vi "Read Panel.vi"(8 "error in (no error)":errorcluster, 11 "Form Configuration in":refnum<class "Form Model Configuration.lvclass">) -> (0 "error out":errorcluster, 2 "Panel.lvlib:Panel.lvclass":refnum<class "Panel.lvclass">, 3 "Form Configuration out":refnum<class "Form Model Configuration.lvclass">)   [LabVIEW 2020]
uses:
  Form Model Configuration.lvclass
  <vilib>/MGI/Panel Manager/Panel/Panel/Panel.lvclass
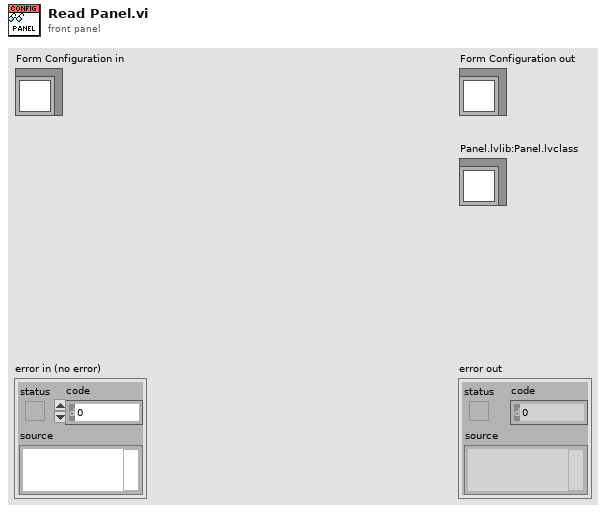
[diagram p1: front panel]
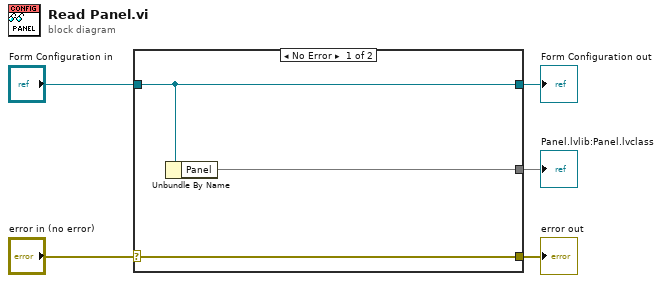
[diagram p0: block diagram]
diagram:
  n1 = case shown="No Error" "error in (no error)" {
    selector: "error in (no error)" -> [w8 w9]
    tunnel: [w8 w9] -> w4
    tunnel: [w7 w10] -> w2
    tunnel: "Form Configuration in" -> [w7 w10]
    tunnel: [w6 _] -> w1
    frame No Error {
      n2 = Unbundle By Name(w7) -> ("Panel"=w6)
    }
    frame Error {
    }
  }
  "error out" <- w4
  "Form Configuration out" <- w2
  "Panel.lvlib:Panel.lvclass" <- w1
